vi "UI.vi"() -> ()   [LabVIEW 2024]
panel:
  in  "Add Button":bool
  in  "Tab Control":T1(tab)
  in  "Request Name":string caption="Name"
  in  "Broadcast Name":string caption="Name"
  in  "Helper Name":string caption="Name"
  in  "Module Name":string caption="Name"
  # "Prove out UI for the concept of VI scripting a module"
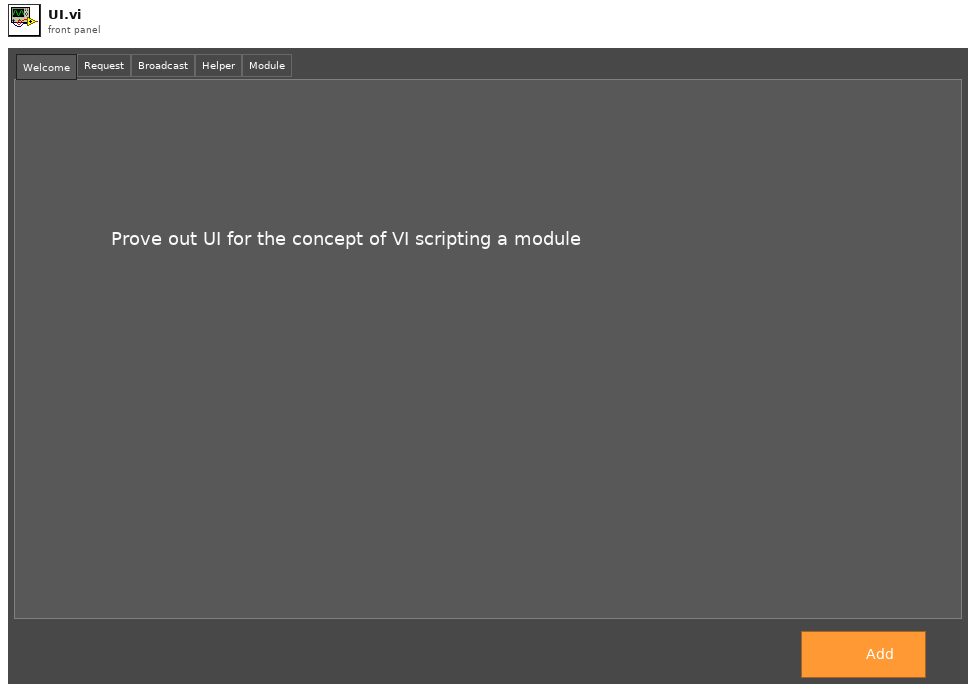
[diagram p1: front panel]
types:
  T1 = enum32{"Welcome", "Request", "Broadcast", "Helper", "Module"}
  T2 = enum32{"Invalid", "Standard", "Closed", "Hidden", "Minimized", "Maximized"}
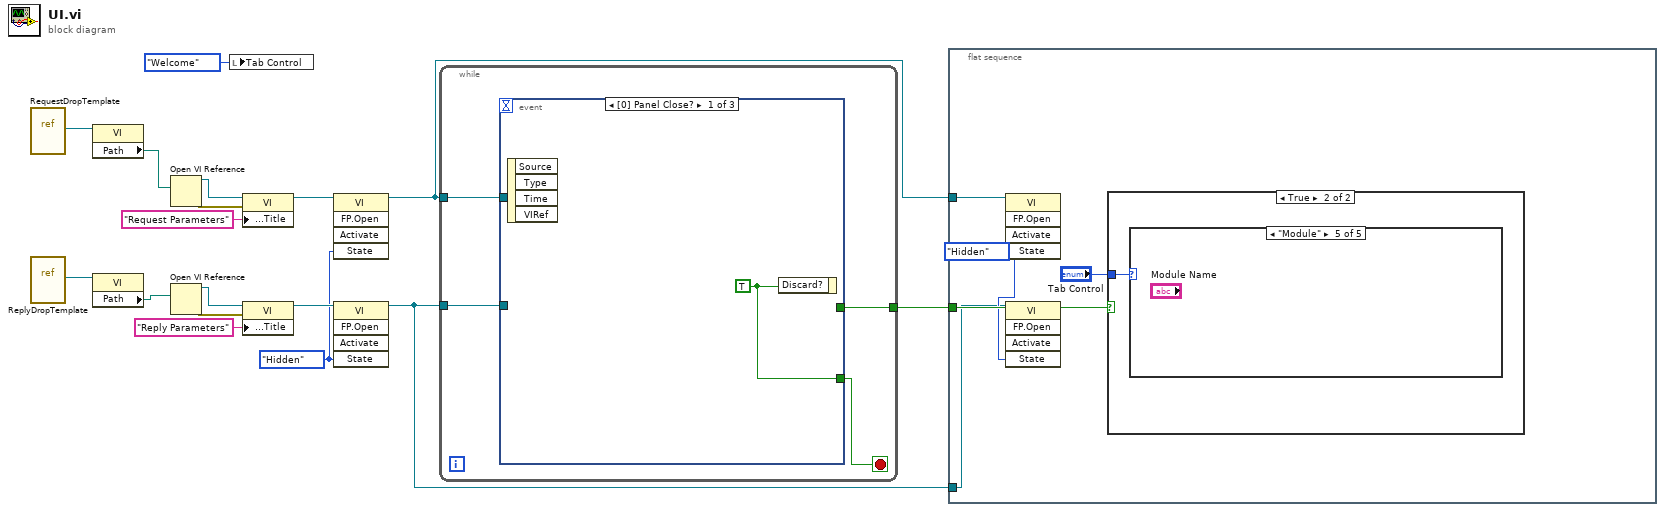
[diagram p0: block diagram]
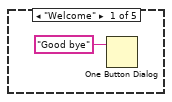
[diagram p3: hidden frame]
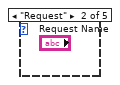
[diagram p4: hidden frame]
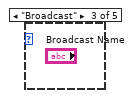
[diagram p5: hidden frame]
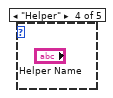
[diagram p6: hidden frame]
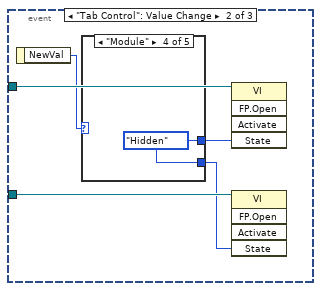
[diagram p7: hidden frame]
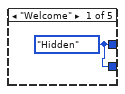
[diagram p8: hidden frame]
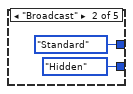
[diagram p9: hidden frame]
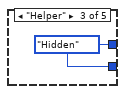
[diagram p10: hidden frame]
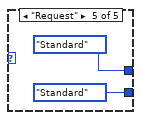
[diagram p11: hidden frame]
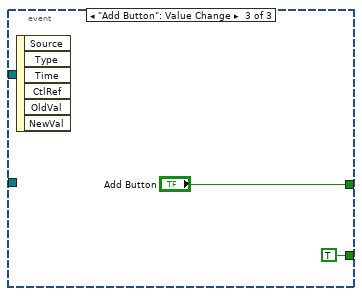
[diagram p12: hidden frame]
diagram:
  w7 = T2."Hidden" ("State")
  n1 = vi-ref "RequestDropTemplate.vi"() -> (w6:refnum<vi>)
  n2 = vi-ref "ReplyDropTemplate.vi"() -> (w4:refnum<vi>)
  n3 = property class="VI"(reference=w6) -> ("Path"=w5:path)  [unwired: 1 in, 2 out]
  n4 = property class="VI"(reference=w4) -> ("Path"=w3:path)  [unwired: 1 in, 2 out]
  n5 = Open VI Reference(vi path=w5) -> (vi reference=w16:refnum<vi>, error out=w17:errorcluster)  [unwired: 5 in]
  n6 = Open VI Reference(vi path=w3) -> (vi reference=w13:refnum<vi>, error out=w12:errorcluster)  [unwired: 5 in]
  n7 = local write "Tab Control"(enum32{"Welcome", "Request", "Broadcast"}."Welcome" ("Tab Control")) -> ()
  n8 = property class="VI"(reference=w16, error in=w17, "Front Panel.Title"="Request Parameters" ("Front Panel Window:Title")) -> (reference out=w8:refnum<vi>)  [unwired: 1 out]
  n9 = property class="VI"(reference=w13, error in=w12, "Front Panel.Title"="Reply Parameters" ("Front Panel Window:Title")) -> (reference out=w9:refnum<vi>)  [unwired: 1 out]
  n10 = invoke class="VI" method="FP.Open"(reference=w8, "State"=w7) -> (reference out=w2:refnum<vi>)  [unwired: 3 in, 4 out]
  n11 = invoke class="VI" method="FP.Open"(reference=w9, "State"=w7) -> (reference out=w1:refnum<vi>)  [unwired: 3 in, 4 out]
  n12 = while {
    tunnel: w1 -> [w19]
    tunnel: w2 -> [w20]
    tunnel: [w18] -> w10
    stop <- w21 stop-if-true
    n13 = event shown="[0] Panel Close?" {
      selector: _ -> [_ _ _]
      dyn-events: _ -> [_ _ _]
      timeout: _ -> [_ _ _]
      tunnel: [w22 _ TRUE] -> w21
      tunnel: w20 -> [_ w27 _]
      tunnel: w19 -> [_ w26 _]
      tunnel: [_ _ "Add Button"] -> w18
      event Panel Close? {
        w22 = TRUE
        n14 = event-data() -> ()  [unwired: 1 in, 4 out]
        n15 = event-data("Discard?"=w22) -> ()  [unwired: 1 in, 1 out]
      }
      event "Tab Control": Value Change {
        n16 = event-data() -> ("NewVal"=w25:T1)  [unwired: 1 in]
        n17 = case shown="\"Module\"" w25 {
          tunnel: [w28 T2."Standard" ("State") w31 w32 T2."Standard" ("State")] -> w24
          tunnel: [w28 T2."Hidden" ("State") w31 w32 T2."Standard" ("State")] -> w23
          frame "Welcome" {
            w28 = T2."Hidden" ("State")
          }
          frame "Broadcast" {
          }
          frame "Helper" {
            w31 = T2."Hidden" ("State")
          }
          frame "Module" {
            w32 = T2."Hidden" ("State")
          }
          frame "Request" {
          }
        }
        n18 = invoke class="VI" method="FP.Open"(reference=w27, "State"=w24) -> ()  [unwired: 3 in, 5 out]
        n19 = invoke class="VI" method="FP.Open"(reference=w26, "State"=w23) -> ()  [unwired: 3 in, 5 out]
      }
      event "Add Button": Value Change {
        n20 = event-data() -> ()  [unwired: 1 in, 6 out]
      }
    }
  }
  n21 = flat-sequence {
    tunnel: w10 -> [w41]
    tunnel: w2 -> [w38]
    tunnel: w1 -> [w37]
    frame #0 {
      w39 = T2."Hidden" ("State")
      n22 = invoke class="VI" method="FP.Open"(reference=w38, "State"=w39) -> ()  [unwired: 3 in, 5 out]
      n23 = invoke class="VI" method="FP.Open"(reference=w37, "State"=w39) -> ()  [unwired: 3 in, 5 out]
      n24 = case shown="True" w41 {
        tunnel: "Tab Control" -> [_ w42]
        frame False {
        }
        frame True {
          n25 = case shown="\"Module\"" w42 {
            frame "Welcome" {
              n26 = One Button Dialog(message="Good bye") -> ()  [unwired: 1 in, 1 out]
            }
            frame "Request" {
            }
            frame "Broadcast" {
            }
            frame "Helper" {
            }
            frame "Module" {
            }
          }
        }
      }
    }
  }
